vi "PollingData.vi"(2 "UnitType":T1(ring)=enum."Power Rider 12", 3 "Ch num 2":u8(ring) items=["Ch 1"]) -> (0 "Array":T2(array[cluster]))   [LabVIEW 2017]
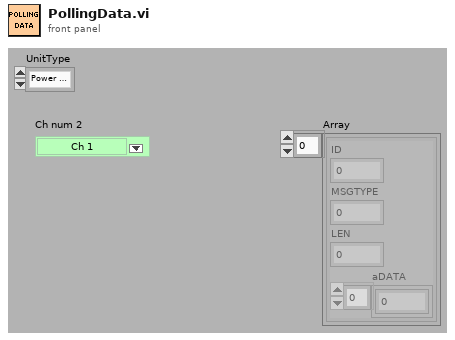
[diagram p1: front panel]
types:
  T1 = enum16{"Single SCB", "Power Rider", "Power Rider&Next10", "HATAL", "DAPH", "Indefinite", "Power Rider 12"}
  T2 = cluster{"ID":u32, "MSGTYPE":u8, "LEN":u8, "aDATA":u8[]}[]
  T3 = cluster{"ID":u32, "MSGTYPE":u8, "LEN":u8, "aDATA":u8[]}
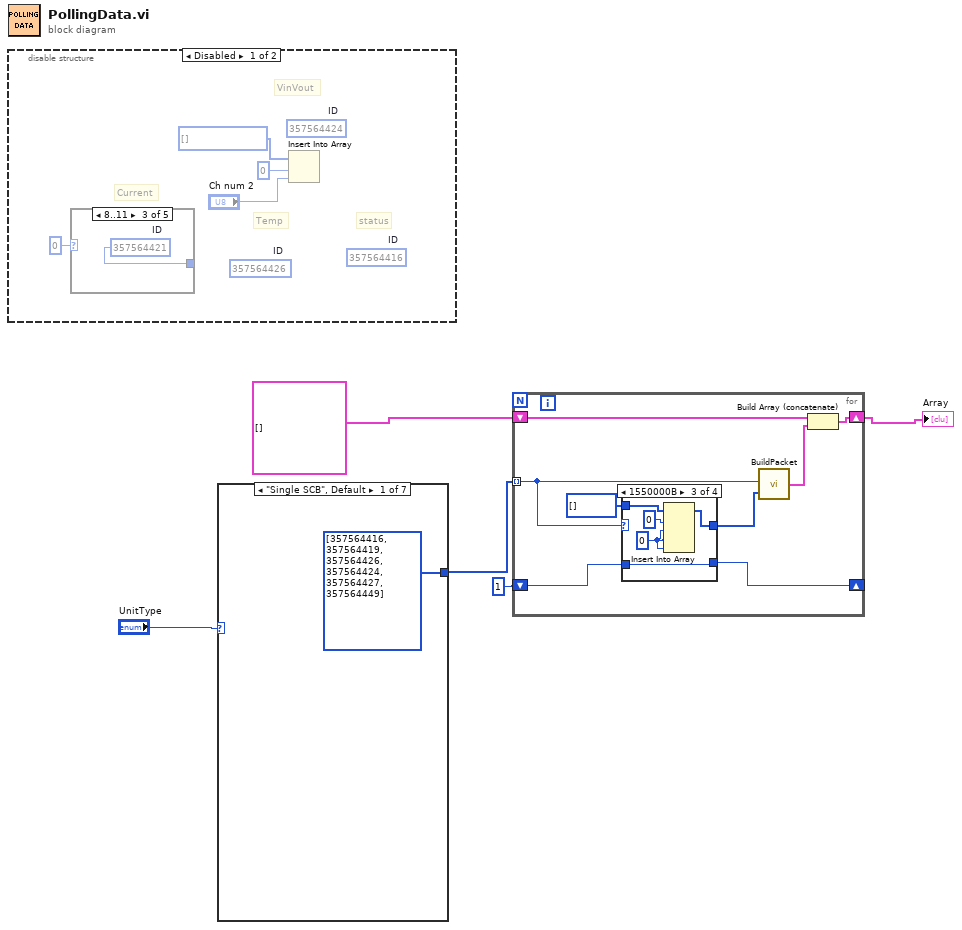
[diagram p0: block diagram]
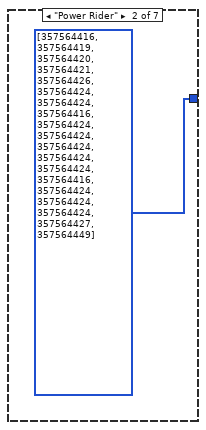
[diagram p2: hidden frame]
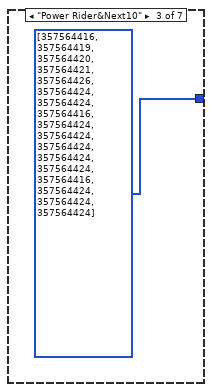
[diagram p3: hidden frame]
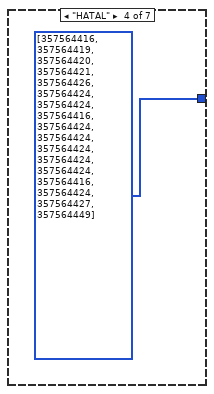
[diagram p4: hidden frame]
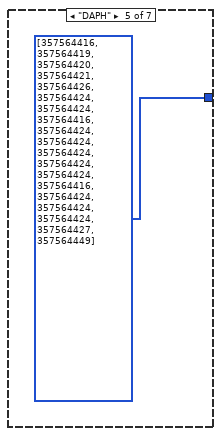
[diagram p5: hidden frame]
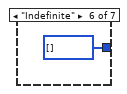
[diagram p6: hidden frame]
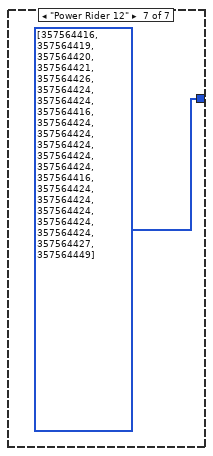
[diagram p7: hidden frame]
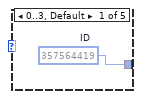
[diagram p8: hidden frame]
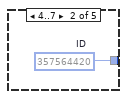
[diagram p9: hidden frame]
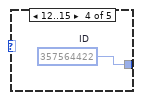
[diagram p10: hidden frame]
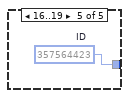
[diagram p11: hidden frame]
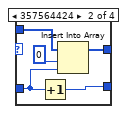
[diagram p14: hidden frame]
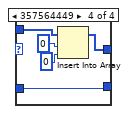
[diagram p15: hidden frame]
diagram:
  n1 = disable-structure shown="Disabled" {
    frame Disabled {
      (unwired) u32 357564424  # ID
      (unwired) u32 357564426  # ID
      (unwired) u32 357564416  # ID
      # "Current"
      # "VinVout"
      # "Temp"
      # "status"
      n2 = case shown="8..11" u8 0 ("Ch num 2") {
        tunnel: [w10 w11 w12 w13 w14] -> _
        frame 0..3, Default {
          w10 = u32 357564419  # ID
        }
        frame 4..7 {
          w11 = u32 357564420  # ID
        }
        frame 8..11 {
          w12 = u32 357564421  # ID
        }
        frame 12..15 {
          w13 = u32 357564422  # ID
        }
        frame 16..19 {
          w14 = u32 357564423  # ID
        }
      }
      n3 = Insert Into Array(array=u8[] [] ("Data 2"), index=0, new element="Ch num 2") -> ()  [unwired: 1 out]
    }
    frame Enabled {
    }
  }
  n4 = case shown="\"Single SCB\", Default" "UnitType" {
    tunnel: [u32[] [357564416, 357564419, 357564426, 357564424, 357564427, 357564449] u32[] [357564416, 357564419, 357564420, 357564421, 357564426, 357564424, 357564424, 357564416, 357564424, 357564424, 357564424, 357564424, 357564424, 357564416, 357564424, 357564424, 357564424, 357564427, 357564449] u32[] [357564416, 357564419, 357564420, 357564421, 357564426, 357564424, 357564424, 357564416, 357564424, 357564424, 357564424, 357564424, 357564424, 357564416, 357564424, 357564424, 357564424] u32[] [357564416, 357564419, 357564420, 357564421, 357564426, 357564424, 357564424, 357564416, 357564424, 357564424, 357564424, 357564424, 357564424, 357564416, 357564424, 357564427, 357564449] u32[] [357564416, 357564419, 357564420, 357564421, 357564426, 357564424, 357564424, 357564416, 357564424, 357564424, 357564424, 357564424, 357564424, 357564416, 357564424, 357564424, 357564424, 357564427, 357564449] u32[] [] u32[] [357564416, 357564419, 357564420, 357564421, 357564426, 357564424, 357564424, 357564416, 357564424, 357564424, 357564424, 357564424, 357564424, 357564416, 357564424, 357564424, 357564424, 357564424, 357564424, 357564427, 357564449]] -> w1
    frame "Single SCB", Default {
    }
    frame "Power Rider" {
    }
    frame "Power Rider&Next10" {
    }
    frame "HATAL" {
    }
    frame "DAPH" {
    }
    frame "Indefinite" {
    }
    frame "Power Rider 12" {
    }
  }
  n5 = for {
    shift-right: [w27] -> w4
    shift-left: T2 [] ("Array") -> [w29]
    tunnel: w1 -> [w22] mode=indexing
    shift-right: [w23] -> _
    shift-left: 1 -> [w24]
    n6 = case shown="1550000B" w22 {
      tunnel: [w31 w36 w41 w46] -> w26
      tunnel: u8[] [] ("Data 2") -> [w31 w35 w40 w45]
      tunnel: w24 -> [w30 w33 w38 w43]
      tunnel: [w30 w32 w38 w43] -> w23
      frame 0, Default {
      }
      frame 357564424 {
        n7 = Increment(x=w33) -> (x+1=w32:i32)
        n8 = Insert Into Array(array=w35, index=0, new element=w33) -> (w36:u8[])
      }
      frame 357564427 {
        w37 = u8 0 ("new element/subarray")
        n9 = Insert Into Array(array=w40, index=0, new element #1=w37, new element #2=w37, new element #3=w37) -> (w41:u8[])
      }
      frame 357564449 {
        n10 = Insert Into Array(array=w45, index=0, new element=u8 0 ("new element/subarray")) -> (w46:u8[])
      }
    }
    n11 = call "BuildPacket.vi"("Data"=w26, "TxID"=w22) -> ("MsgTX 2"=w28:T3)
    n12 = Build Array (concatenate)(w29, w28) -> (w27:T2)
  }
  "Array" <- w4
